vi "HEWH General Start End Draw.vi"(7 "Index Type":T1, 8 "error in (no error)":errorcluster, 10 "Draw Start":i32, 11 "UEF Calculated Values in":T2 {"Data Indexes"."15 sec after Draw Index" format="%#.2f"; "Data Indexes"."15 sec after Draw Timestamp" format="%#.2f"; "Data Indexes"."Test Start Timestamp" format="%.2f"; "Data Indexes"."Test End Timestamp" format="%.2f"; "Data Indexes"."T0 Timestamp" format="%.2f"; "Data Indexes"."Tsf Timestamp" format="%.2f"; "Data Indexes"."Tsu0 Timestamp" format="%.2f"; "Data Indexes"."Tmax1 Timestamp" format="%.2f"; "Data Indexes"."Draw Index Timestamp" format="%#.2f"; "Data Indexes"."Non-Draw Timestamp" format="%#.2f"; "Data Indexes"."Heating Timestamp" format="%#.2f"; "Data Indexes"."Start Energy (BTU-Gas)" format="%.6f"; "Data Indexes"."Start Watt Hours" format="%.6f"; "Static Data"."V - Volume of Wh (True)" format="%.5f"; "Static Data"."T-Ambinet Nominal (°F)" format="%.5f"; "Static Data"."T-Inlet Setpoint (°F)" format="%.5f"; "Static Data"."T-Wh Setpoint (°F)" format="%.5f"; "Sampled Data"."Qe (Wh)" format="%.5f"; "Sampled Data"."Tau stby2 (hr)" format="%.5f"; "Sampled Data"."Tastby2 (°F)" format="%.5f"; "Sampled Data"."Qf (BTU)" format="%.5f"; "Sampled Data"."Qe (BTU)" format="%.5f"; "Sampled Data"."Tmax1 (°F)" format="%.5f"; "Sampled Data"."T0 (°F)" format="%.5f"; "Sampled Data"."Qr (BTU)" format="%.5f"; "Sampled Data"."T 24(°F)" format="%.5f"; "Sampled Data"."T astby(°F)" format="%.5f"; "Sampled Data"."T tstby(°F)" format="%.5f"; "Sampled Data"."T su0(°F)" format="%.5f"; "Sampled Data"."T suf(°F)" format="%.5f"; "Sampled Data"."Tau stby_1 (hr)" format="%.5f"; "Sampled Data"."Qsuf (BTU)" format="%.5f"; "Sampled Data"."Qsu0 (BTU)" format="%.5f"; "Calculated Values"."Draw Bonus Volume (gal)" format="%.6f"; "Calculated Values"."Adjustment Factor" format="%.6f"; "Calculated Values"."T*avg_del(n-1)" format="%.6f"; "Calculated Values"."T*min(n-1)" format="%.6f"; "Calculated Values"."T*avg_del(n)" format="%.6f"; "Calculated Values"."Vn" format="%.6f"; "Calculated Values"."Qdm (BTU)" format="%.6f"; "Calculated Values"."QHWD (BTU)" format="%.6f"; "Calculated Values"."QHW (BTU)" format="%.6f"; "Calculated Values"."UEF" format="%.6f"; "Calculated Values"."QHW67 (BTU)" format="%.6f"; "Calculated Values"."Qda (BTU)" format="%.6f"; "Calculated Values"."Qd (BTU)" format="%.6f"; "Calculated Values"."Q (BTU)" format="%.6f"; "Calculated Values"."UA (BTU/(hr*F))" format="%.6f"; "Calculated Values"."Qhr (BTU/hr)" format="%.6f"; "Calculated Values"."Qstby (BTU)" format="%.6f"; "Calculated Values"."nu_r" format="%.6f"; "Calculated Values"."CpUEF (BTU/(lb*F))" format="%.6f"; "Calculated Values"."rho_nu (lb/gal)" format="%.6f"; "Calculated Values"."V1- Vol (Gal)" format="%.6f"; "Calculated Values"."M cluster mass removed (lb)" format="%.6f"; "Calculated Values"."Cp theoretical (BTU/(lbm °F))" format="%.6f"; "Calculated Values"."Tin1 - Mean Inlet 1st Cluster (°F)" format="%.6f"; "Calculated Values"."Tdel1-Mean Outlet 1st Cluster(°F)" format="%.6f"; "Calculated Values"."Cp 24 (BTU/(lb*F))" format="%.6f"; "Calculated Values"."Cp standby (BTU/(lb*F))" format="%.6f"; "Calculated Values"."Cp2 (BTU/(lb*F))" format="%.6f"; "Calculated Values"."Cp1 (BTU/(lb*F))" format="%.6f"; "Calculated Values"."rho 24 (lb/gal)" format="%.6f"; "Calculated Values"."rho standby (lb/gal)" format="%.6f"; "Calculated Values"."rho 2 (lb/gal)" format="%.6f"; "Calculated Values"."Density of cold water All (lbm/gal)" format="%#.3g"; "Calculated Values"."CpHW (BTU/(lbm °F))" format="%#.3g"; "Calculated Values"."Density of hot water All (lbm/gal)" format="%#.3g"; "Calculated Values"."Mass of water All (lbm)" format="%#.3f"}) -> (0 "error out":errorcluster, 2 "End Index":i32, 3 "UEF Calculated Values Output":T2 {"Data Indexes"."15 sec after Draw Index" format="%#.2f"; "Data Indexes"."15 sec after Draw Timestamp" format="%#.2f"; "Data Indexes"."Test Start Timestamp" format="%.2f"; "Data Indexes"."Test End Timestamp" format="%.2f"; "Data Indexes"."T0 Timestamp" format="%.2f"; "Data Indexes"."Tsf Timestamp" format="%.2f"; "Data Indexes"."Tsu0 Timestamp" format="%.2f"; "Data Indexes"."Tmax1 Timestamp" format="%.2f"; "Data Indexes"."Draw Index Timestamp" format="%#.2f"; "Data Indexes"."Non-Draw Timestamp" format="%#.2f"; "Data Indexes"."Heating Timestamp" format="%#.2f"; "Data Indexes"."Start Energy (BTU-Gas)" format="%.6f"; "Data Indexes"."Start Watt Hours" format="%.6f"; "Static Data"."V - Volume of Wh (True)" format="%.5f"; "Static Data"."T-Ambinet Nominal (°F)" format="%.5f"; "Static Data"."T-Inlet Setpoint (°F)" format="%.5f"; "Static Data"."T-Wh Setpoint (°F)" format="%.5f"; "Sampled Data"."Qe (Wh)" format="%.5f"; "Sampled Data"."Tau stby2 (hr)" format="%.5f"; "Sampled Data"."Tastby2 (°F)" format="%.5f"; "Sampled Data"."Qf (BTU)" format="%.5f"; "Sampled Data"."Qe (BTU)" format="%.5f"; "Sampled Data"."Tmax1 (°F)" format="%.5f"; "Sampled Data"."T0 (°F)" format="%.5f"; "Sampled Data"."Qr (BTU)" format="%.5f"; "Sampled Data"."T 24(°F)" format="%.5f"; "Sampled Data"."T astby(°F)" format="%.5f"; "Sampled Data"."T tstby(°F)" format="%.5f"; "Sampled Data"."T su0(°F)" format="%.5f"; "Sampled Data"."T suf(°F)" format="%.5f"; "Sampled Data"."Tau stby_1 (hr)" format="%.5f"; "Sampled Data"."Qsuf (BTU)" format="%.5f"; "Sampled Data"."Qsu0 (BTU)" format="%.5f"; "Calculated Values"."Draw Bonus Volume (gal)" format="%.6f"; "Calculated Values"."Adjustment Factor" format="%.6f"; "Calculated Values"."T*avg_del(n-1)" format="%.6f"; "Calculated Values"."T*min(n-1)" format="%.6f"; "Calculated Values"."T*avg_del(n)" format="%.6f"; "Calculated Values"."Vn" format="%.6f"; "Calculated Values"."Qdm (BTU)" format="%.6f"; "Calculated Values"."QHWD (BTU)" format="%.6f"; "Calculated Values"."QHW (BTU)" format="%.6f"; "Calculated Values"."UEF" format="%.6f"; "Calculated Values"."QHW67 (BTU)" format="%.6f"; "Calculated Values"."Qda (BTU)" format="%.6f"; "Calculated Values"."Qd (BTU)" format="%.6f"; "Calculated Values"."Q (BTU)" format="%.6f"; "Calculated Values"."UA (BTU/(hr*F))" format="%.6f"; "Calculated Values"."Qhr (BTU/hr)" format="%.6f"; "Calculated Values"."Qstby (BTU)" format="%.6f"; "Calculated Values"."nu_r" format="%.6f"; "Calculated Values"."CpUEF (BTU/(lb*F))" format="%.6f"; "Calculated Values"."rho_nu (lb/gal)" format="%.6f"; "Calculated Values"."V1- Vol (Gal)" format="%.6f"; "Calculated Values"."M cluster mass removed (lb)" format="%.6f"; "Calculated Values"."Cp theoretical (BTU/(lbm °F))" format="%.6f"; "Calculated Values"."Tin1 - Mean Inlet 1st Cluster (°F)" format="%.6f"; "Calculated Values"."Tdel1-Mean Outlet 1st Cluster(°F)" format="%.6f"; "Calculated Values"."Cp 24 (BTU/(lb*F))" format="%.6f"; "Calculated Values"."Cp standby (BTU/(lb*F))" format="%.6f"; "Calculated Values"."Cp2 (BTU/(lb*F))" format="%.6f"; "Calculated Values"."Cp1 (BTU/(lb*F))" format="%.6f"; "Calculated Values"."rho 24 (lb/gal)" format="%.6f"; "Calculated Values"."rho standby (lb/gal)" format="%.6f"; "Calculated Values"."rho 2 (lb/gal)" format="%.6f"; "Calculated Values"."Density of cold water All (lbm/gal)" format="%#.3g"; "Calculated Values"."CpHW (BTU/(lbm °F))" format="%#.3g"; "Calculated Values"."Density of hot water All (lbm/gal)" format="%#.3g"; "Calculated Values"."Mass of water All (lbm)" format="%#.3f"})   [LabVIEW 2023]
uses:
  Type Definitions/UEF Constants.ctl
  Type Definitions/HEWH Draw Stats.ctl
  Type Definitions/HEWH FHR Draw Type.ctl
  Type Definitions/FHR Bins.ctl
  Type Definitions/HEWH Meter Type.ctl
  Type Definitions/HEWH Index Type.ctl
panel:
  out "subarray":dbl[](array[numeric])
  # "FHR"
  # "FHR"
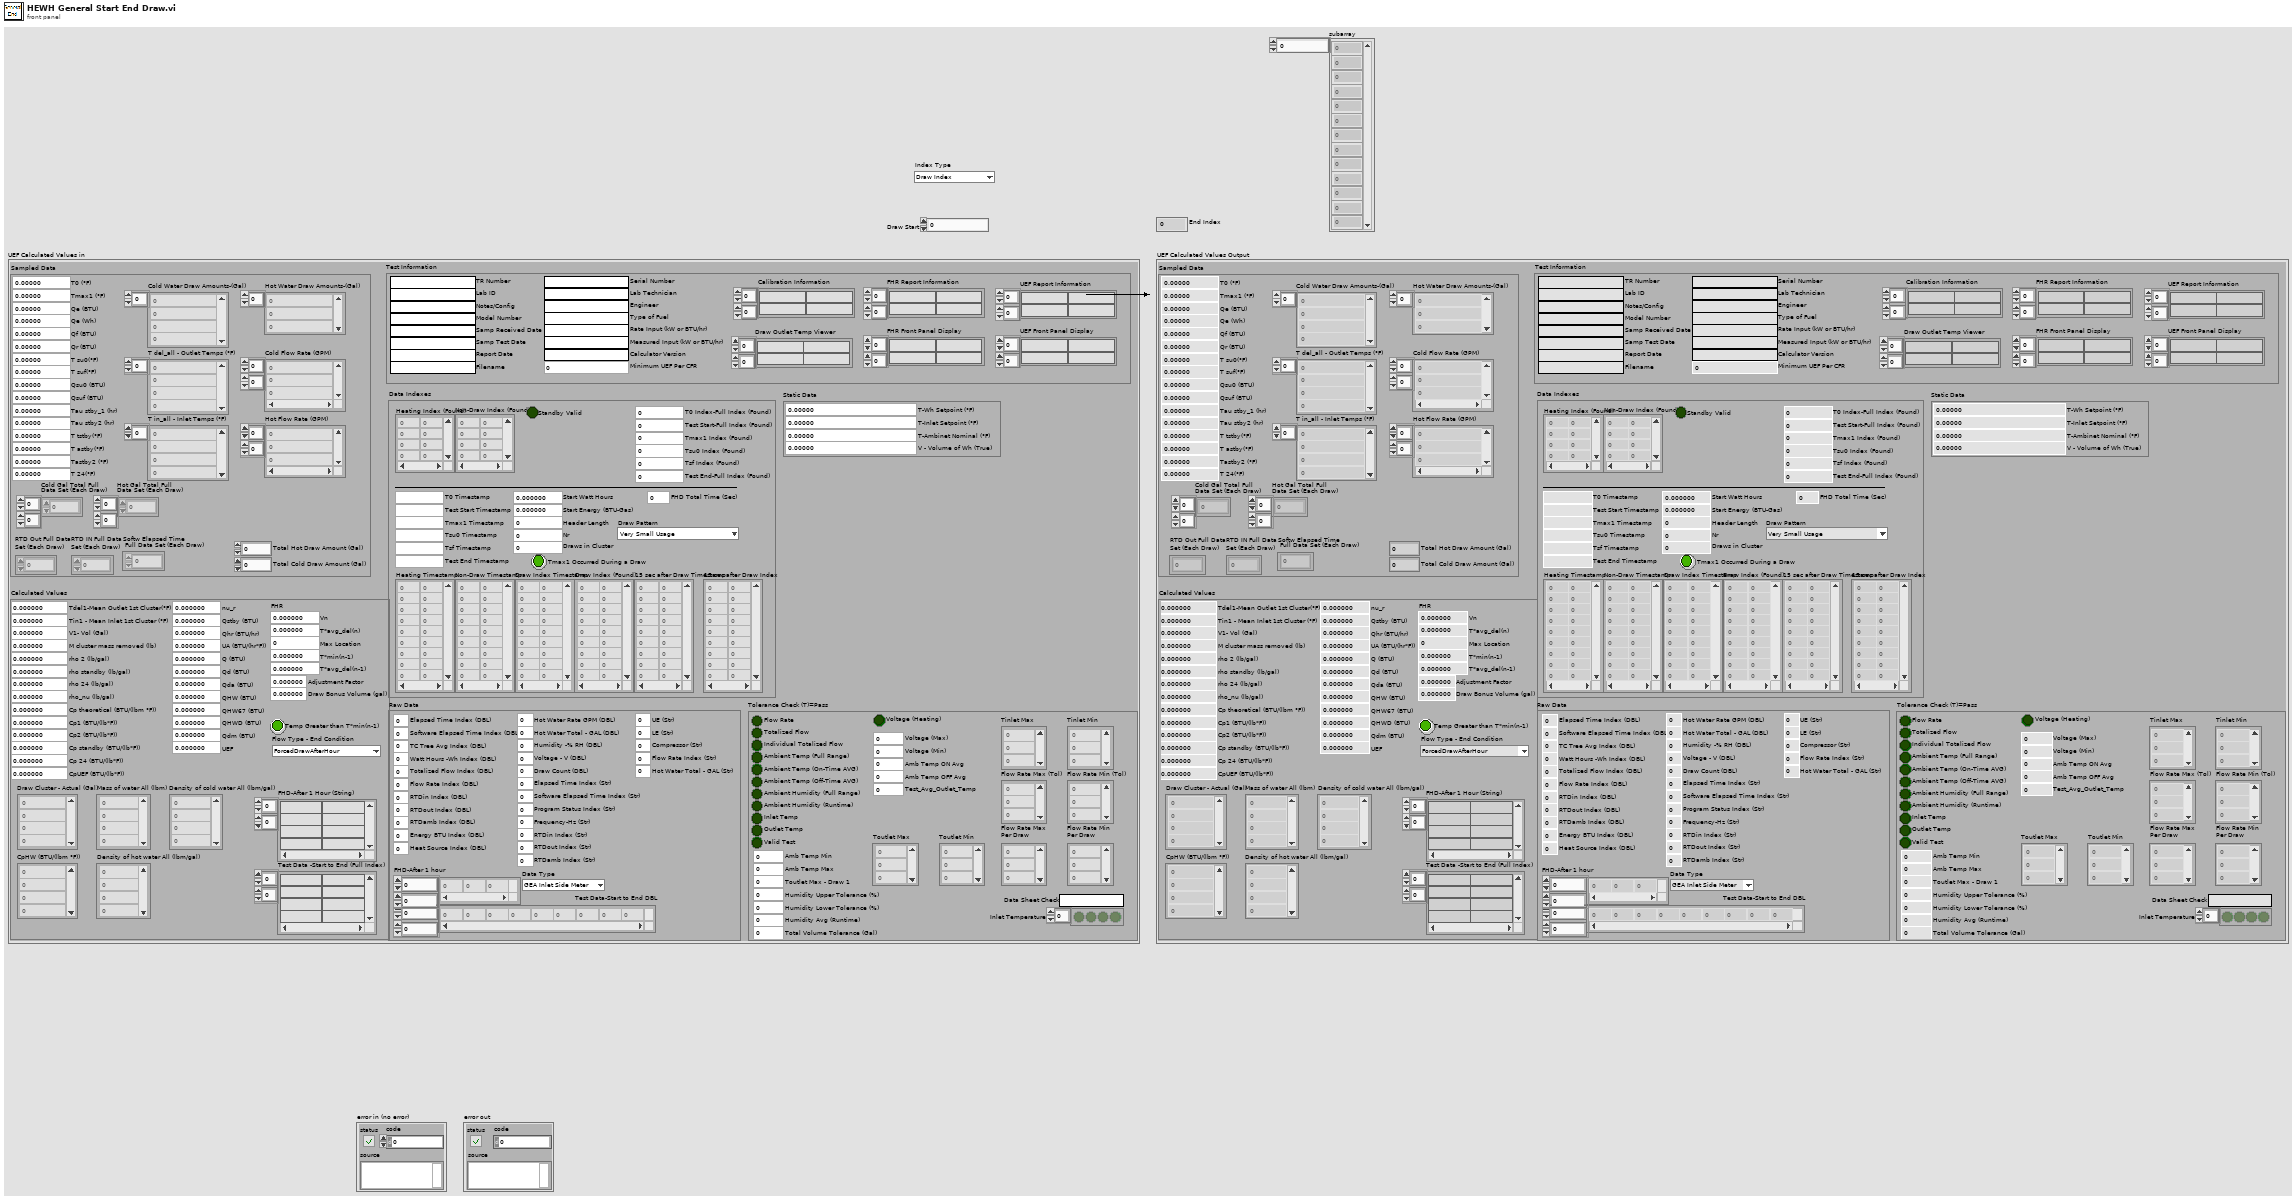
[diagram p1: front panel]
types:
  T1 = typedef "HEWH Index Type.ctl" = enum16{"Draw Index", "Heating Index", "Temp Based (FHD)"}
  T2 = typedef "UEF Constants.ctl" = cluster{"Calculated Values":T3, "Sampled Data":cluster{"Cold Water Draw Amounts-(Gal)":dbl[], "T del_all - Outlet Temps (°F)":dbl[], "T in_all - Inlet Temps (°F)":dbl[], "Qsu0 (BTU)":dbl, "Qsuf (BTU)":dbl, "Tau stby_1 (hr)":dbl, "T suf(°F)":dbl, "T su0(°F)":dbl, "T tstby(°F)":dbl, "T astby(°F)":dbl, "T 24(°F)":dbl, "Qr (BTU)":dbl, "T0 (°F)":dbl, "Tmax1 (°F)":dbl, "Qe (BTU)":dbl, "Qf (BTU)":dbl, "Tastby2 (°F)":dbl, "RTD Out Full Data\nSet (Each Draw)":dbl[][], "RTD IN Full Data\nSet (Each Draw)":dbl[][], "Tau stby2 (hr)":dbl, "Hot Water Draw Amounts-(Gal)":dbl[], "Cold Flow Rate (GPM)":dbl[][], "Hot Flow Rate (GPM)":dbl[][], "Softw Elapsed Time\n Full Data Set (Each Draw)":dbl[][], "Cold Gal Total Full\nData Set (Each Draw)":dbl[][], "Total Hot Draw Amount (Gal) ":dbl, "Total Cold Draw Amount (Gal)":dbl, "Qe (Wh)":dbl, "Hot Gal Total Full\nData Set (Each Draw)":dbl[][]}, "Static Data":cluster{"T-Wh Setpoint (°F)":dbl, "T-Inlet Setpoint (°F)":dbl, "T-Ambinet Nominal (°F)":dbl, "V - Volume of Wh (True)":dbl}, "Data Indexes":cluster{"Test Start-Full Index (Found)":i32, "Header Length":i32, "Draw Index (Found)":i32[][], "Nr":i32, "Start Watt Hours":dbl, "Tsu0 Index (Found)":i32, "Tsf Index (Found)":i32, "Start Energy (BTU-Gas)":dbl, "Draws in Cluster":i32, "T0 Index-Full Index (Found)":i32, "Non-Draw Index (Found)":i32[][], "Tmax1 Index (Found)":i32, "Test End-Full Index (Found)":i32, "Heating Index (Found)":i32[][], "Heating Timestamp":dbl[][], "Non-Draw Timestamp":dbl[][], "Draw Index Timestamp":dbl[][], "Tmax1 Timestamp":dbl, "Tsu0 Timestamp":dbl, "Tsf Timestamp":dbl, "T0 Timestamp":dbl, "Test End Timestamp":dbl, "Test Start Timestamp":dbl, "15 sec after Draw Timestamp":dbl[][], "15 sec after Draw Index":dbl[][], "Tmax1 Occurred During a Draw":bool, "FHD Total Time (Sec)":dbl, "Draw Pattern":T5, "Standby Valid":bool}, "Raw Data":cluster{"Elapsed Time Index (DBL)":i32, "Software Elapsed Time Index (DBL)":i32, "TC Tree Avg Index (DBL)":i32, "Watt Hours -Wh Index (DBL)":i32, "Energy BTU Index (DBL)":i32, "Totalized Flow Index (DBL)":i32, "Flow Rate Index (DBL)":i32, "Program Status Index (Str)":i32, "RTDin Index (DBL)":i32, "RTDout Index (DBL)":i32, "RTDamb Index (DBL)":i32, "Test Data-Start to End DBL":dbl[][], "Data Type":T6, "Heat Source Index (DBL)":i32, "Hot Water Rate GPM (DBL)":i32, "Hot Water Total - GAL (DBL)":i32, "FHD-After 1 hour":dbl[][], "Humidity -% RH (DBL)":i32, "Voltage - V (DBL)":i32, "Draw Count (DBL)":i32, "Elapsed Time Index (Str)":i32, "Software Elapsed Time Index (Str)":i32, "Frequency-Hz (Str)":i32, "RTDin Index (Str)":i32, "RTDout Index (Str)":i32, "RTDamb Index (Str)":i32, "UE (Str)":i32, "LE (Str)":i32, "Compressor (Str)":i32, "Flow Rate Index (Str)":i32, "Hot Water Total - GAL (Str)":i32}, "Tolerance Check (T)=Pass":cluster{"Flow Rate":bool, "Totalized Flow":bool, "Ambient Temp (Full Range)":bool, "Ambient Humidity (Full Range)":bool, "Inlet Temp":bool, "Outlet Temp":bool, "Valid Test":bool, "Individual Totalized Flow":bool, "Data Sheet Check":string, "Inlet Temperature":bool[], "Tinlet Max":dbl[], "Tinlet Min":dbl[], "Flow Rate Max (Tol)":dbl[], "Flow Rate Min (Tol)":dbl[], "Amb Temp Max":dbl, "Amb Temp Min":dbl, "Toutlet Max - Draw 1":dbl, "Humidity Upper Tolerance (%)":dbl, "Total Volume Tolerance (Gal)":dbl, "Humidity Lower Tolerance (%)":dbl, "Flow Rate Max\nPer Draw":dbl[], "Flow Rate Min\nPer Draw":dbl[], "Ambient Humidity (Runtime)":bool, "Humidity Avg (Runtime)":dbl, "Ambient Temp (On-Time AVG)":bool, "Ambient Temp (Off-Time AVG)":bool, "Amb Temp OFF Avg":dbl, "Amb Temp ON Avg":dbl, "Voltage (Heating)":bool, "Voltage (Min)":dbl, "Voltage (Max)":dbl, "Toutlet Max":dbl[], "Toutlet Min":dbl[], "Test_Avg_Outlet_Temp":dbl}, "Test Information":cluster{"TR Number":string, "Lab ID":string, "Notes/Config":string, "Model Number":string, "Serial Number":string, "Lab Technician":string, "Engineer":string, "Type of Fuel":string, "Samp Received Date":string, "Samp Test Date":string, "Report Date":string, "Rate Input (kW or BTU/hr)":string, "Measured Input (kW or BTU/hr)":string, "Filename":string, "Calibration Information":string[][], "Calculator Version":string, "Minimum UEF Per CFR":dbl, "UEF Report Information":string[][], "FHR Report Information":string[][], "FHR Front Panel Display":string[][], "UEF Front Panel Display":string[][], "Draw Outlet Temp Viewer":string[][]}}
  T3 = typedef "HEWH Draw Stats.ctl" = cluster{"Draw Cluster - Actual (Gal)":dbl[], "Mass of water All (lbm)":dbl[], "Density of hot water All (lbm/gal)":dbl[], "CpHW (BTU/(lbm °F))":dbl[], "rho 2 (lb/gal)":dbl, "rho standby (lb/gal)":dbl, "rho 24 (lb/gal)":dbl, "Cp1 (BTU/(lb*F))":dbl, "Cp2 (BTU/(lb*F))":dbl, "Cp standby (BTU/(lb*F))":dbl, "Cp 24 (BTU/(lb*F))":dbl, "nu_r":dbl, "Qstby (BTU)":dbl, "Qhr (BTU/hr)":dbl, "UA (BTU/(hr*F))":dbl, "Q (BTU)":dbl, "Qd (BTU)":dbl, "Qda (BTU)":dbl, "QHW67 (BTU)":dbl, "UEF":dbl, "Tdel1-Mean Outlet 1st Cluster(°F)":dbl, "Tin1 - Mean Inlet 1st Cluster (°F)":dbl, "Cp theoretical (BTU/(lbm °F))":dbl, "M cluster mass removed (lb)":dbl, "V1- Vol (Gal)":dbl, "Test Data -Start to End (Full Index)":string[][], "rho_nu (lb/gal)":dbl, "Density of cold water All (lbm/gal)":dbl[], "CpUEF (BTU/(lb*F))":dbl, "QHW (BTU)":dbl, "QHWD (BTU)":dbl, "Qdm (BTU)":dbl, "FHD-After 1 Hour (String)":string[][], "Vn":dbl, "T*avg_del(n)":dbl, "Max Location":i32, "T*min(n-1)":dbl, "T*avg_del(n-1)":dbl, "Temp Greater than T*min(n-1)":bool, "Adjustment Factor":dbl, "Draw Bonus Volume (gal)":dbl, "Flow Type - End Condition":T4}
  T4 = typedef "HEWH FHR Draw Type.ctl" = enum16{"ForcedDrawAfterHour", "HeatingCutoffBeforeHour"}
  T5 = typedef "FHR Bins.ctl" = enum16{"Very Small Usage", "Low Usage", "Medium Usage", "High Usage", "Undefined"}
  T6 = typedef "HEWH Meter Type.ctl" = enum16{"GEA Inlet Side Meter", "GEA Outlet Side Meter", "CSA Inlet Side Meter"}
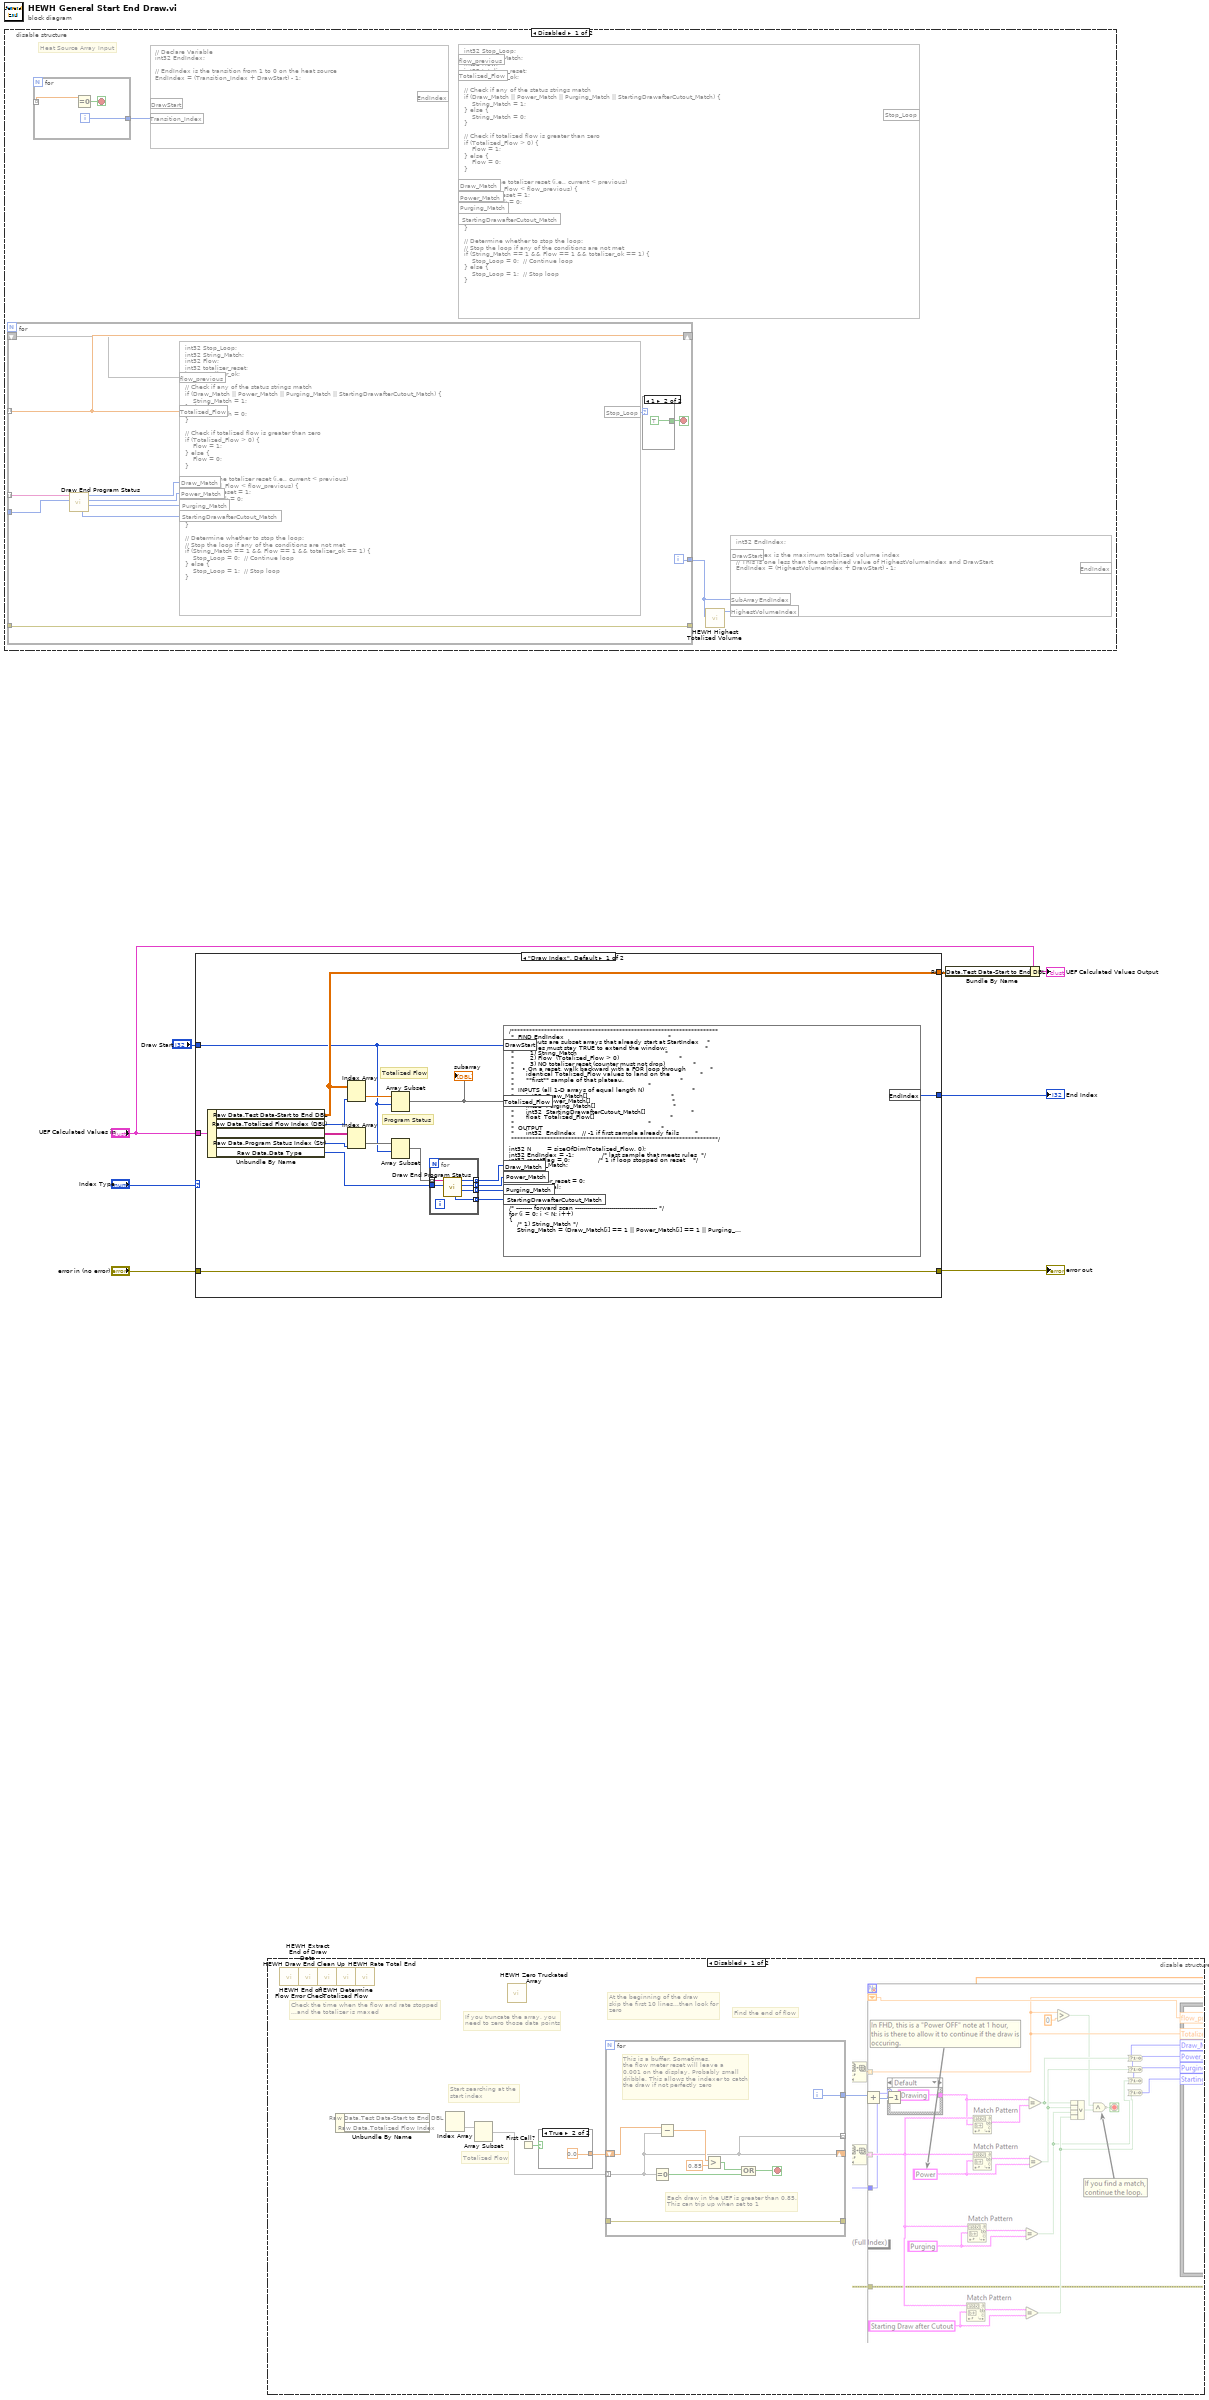
[diagram p0: block diagram]
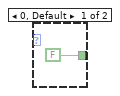
[diagram p2: hidden frame]
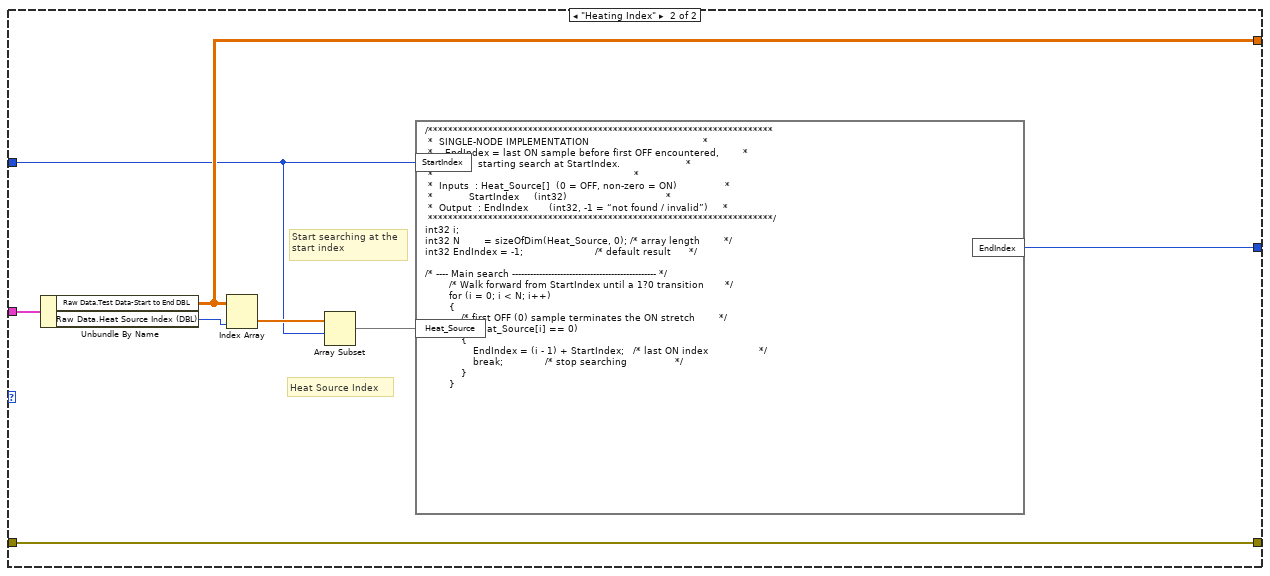
[diagram p6: hidden frame]
diagram:
  n1 = disable-structure shown="Disabled" {
    frame Disabled {
      # "Heat Source Array Input"
      n2 = for {
        tunnel: [w23] -> w9
        tunnel: _ -> [w20] mode=indexing
        tunnel: _ -> [w22]
        tunnel: [w22] -> _
        tunnel: _ -> [w21]
        tunnel: _ -> [w13] mode=indexing
        shift-right: [w13] -> _
        shift-left: _ -> [w12]
        i -> [w23]
        stop <- w14 stop-if-true
        n3 = call "Draw End Program Status.vi"("Data Type"=w21, "Program Status String"=w20) -> ("Purging_Match"=w18:i16, "Power_Match"=w16:i16, "Draw_Match"=w19:i16, "StartingDrawafterCutout_Match"=w17:i16)  [unwired: 6 in]
        n4 = formula code="int32 Stop_Loop;\nint32 String_Match;\nint32 Flow;\nint32 totalizer_reset;\nint32 totalizer_ok;\n\n// Check if any of the status strings match\nif (Draw_Match || Power_Match || Purging_Match || StartingDrawafterCutout_Match) {\n    String_Match = 1;\n} else {\n    String_Match = 0;\n}\n\n// Check if totalized flow is greater than zero\nif (Totalized_Flow > 0) {\n    Flow = 1;\n} else {\n    Flow = 0;\n}\n\n// Check if the totalizer reset (i.e., current < previous)\nif (Totalized_Flow < flow_previous) {\n    totalizer_reset = 1;\n    totalizer_ok = 0;\n} else {\n    totalizer_reset = 0;\n    totalizer_ok = 1;\n}\n\n// Determine whether to stop the loop:\n// Stop the loop if any of the conditions are not met\nif (String_Match == 1 && Flow == 1 && totalizer_ok == 1) {\n    Stop_Loop = 0;  // Continue loop\n} else {\n    Stop_Loop = 1;  // Stop loop\n}"("Draw_Match"=w19, "Power_Match"=w16, "Purging_Match"=w18, "StartingDrawafterCutout_Match"=w17, "Totalized_Flow"=w13, "flow_previous"=w12) -> ("Stop_Loop"=w15:i32)
        n5 = case shown="1" w15 {
          tunnel: [FALSE TRUE] -> w14
          frame 0, Default {
          }
          frame 1 {
          }
        }
      }
      n6 = for {
        tunnel: _ -> [w28] mode=indexing
        tunnel: [w26] -> w11
        i -> [w26]
        stop <- w27 stop-if-true
        n7 = Equal To 0?(x=w28) -> (x = 0?=w27:bool)
      }
      n8 = formula code="// Declare Variable\nint32 EndIndex;\n\n// EndIndex is the transition from 1 to 0 on the heat source\nEndIndex = (Transition_Index + DrawStart) - 1;"("Transition_Index"=w11) -> ()  [unwired: 1 in, 1 out]
      n9 = formula code="int32 Stop_Loop;\nint32 String_Match;\nint32 Flow;\nint32 totalizer_reset;\nint32 totalizer_ok;\n\n// Check if any of the status strings match\nif (Draw_Match || Power_Match || Purging_Match || StartingDrawafterCutout_Match) {\n    String_Match = 1;\n} else {\n    String_Match = 0;\n}\n\n// Check if totalized flow is greater than zero\nif (Totalized_Flow > 0) {\n    Flow = 1;\n} else {\n    Flow = 0;\n}\n\n// Check if the totalizer reset (i.e., current < previous)\nif (Totalized_Flow < flow_previous) {\n    totalizer_reset = 1;\n    totalizer_ok = 0;\n} else {\n    totalizer_reset = 0;\n    totalizer_ok = 1;\n}\n\n// Determine whether to stop the loop:\n// Stop the loop if any of the conditions are not met\nif (String_Match == 1 && Flow == 1 && totalizer_ok == 1) {\n    Stop_Loop = 0;  // Continue loop\n} else {\n    Stop_Loop = 1;  // Stop loop\n}"() -> ()  [unwired: 6 in, 1 out]
      n10 = call "HEWH Highest Totalized Volume.vi"("Sub Array End Index in"=w9) -> ("Highest Volume Index"=w10:i32)  [unwired: 9 in, 1 out]
      n11 = formula code="int32 EndIndex;\n\n// EndIndex is the maximum totalized volume index\n// This is one less than the combined value of HighestVolumeIndex and DrawStart\nEndIndex = (HighestVolumeIndex + DrawStart) - 1;"("HighestVolumeIndex"=w10, "SubArrayEndIndex"=w9) -> ()  [unwired: 1 in, 1 out]
    }
    frame Enabled {
    }
  }
  n12 = case shown="\"Draw Index\", Default" "Index Type" {
    tunnel: "UEF Calculated Values in" -> [w45 w59]
    tunnel: [w39 w57] -> w2
    tunnel: "Draw Start" -> [w31 w54]
    tunnel: "error in (no error)" -> [w29 w56]
    tunnel: [w29 w56] -> w1
    tunnel: [w30 w52] -> w3
    frame "Draw Index", Default {
      # "Program Status"
      # "Totalized Flow"
      n13 = Unbundle By Name(w45) -> ("Raw Data.Test Data-Start to End DBL"=w39:dbl[][], "Raw Data.Totalized Flow Index (DBL)"=w40:i32, "Calculated Values.Test Data -Start to End (Full Index)"=w42:string[][], "Raw Data.Program Status Index (Str)"=w41:i32, "Raw Data.Data Type"=w37:T6)
      n14 = Index Array(array=w39, index (col)=w40) -> (element=w44:dbl[])  [unwired: 1 in]
      n15 = Index Array(array=w42, index (col)=w41) -> (element=w43:string[])  [unwired: 1 in]
      n16 = Array Subset(array=w44, index=w31) -> (w36:dbl[])  [unwired: 1 in]
      "subarray" <- w36
      n17 = Array Subset(array=w43, index=w31) -> (w38:string[])  [unwired: 1 in]
      n18 = for {
        tunnel: w38 -> [w51] mode=indexing
        tunnel: w37 -> [w50]
        tunnel: [w49] -> w35 mode=indexing
        tunnel: [w48] -> w34 mode=indexing
        tunnel: [w47] -> w33 mode=indexing
        tunnel: [w46] -> w32 mode=indexing
        n19 = call "Draw End Program Status.vi"("Data Type"=w50, "Program Status String"=w51) -> ("Purging_Match"=w47:i16, "Power_Match"=w48:i16, "Draw_Match"=w49:i16, "StartingDrawafterCutout_Match"=w46:i16)  [unwired: 6 in]
      }
      n20 = formula code="/*********************************************************************\n *  FIND EndIndex                                                    *\n *    • Inputs are subset arrays that already start at StartIndex    *\n *    • Rules must stay TRUE to extend the window:                   *\n *        1) String_Match                                            *\n *        2) Flow  (Totalized_Flow > 0)                              *\n *        3) NO totalizer reset (counter must not drop)              *\n *    • On a reset, walk backward with a FOR loop through            *\n *      identical Totalized_Flow values to land on the               *\n *      **first** sample of that plateau.                            *\n *                                                                   *\n *  INPUTS (all 1-D arrays of equal length N)                        *\n *      int32  Draw_Match[]                                          *\n *      int32  Power_Match[]                                         *\n *      int32  Purging_Match[]                                       *\n *      int32  StartingDrawafterCutout_Match[]                       *\n *      float  Totalized_Flow[]                                      *\n *                                                                   *\n *  OUTPUT                                                           *\n *      int32  EndIndex   // -1 if first sample already fails        *\n *********************************************************************/\n\nint32 N        = sizeOfDim(Totalized_Flow, 0);\nint32 EndIndex = -1;              /* last sample that meets rules  */\nint32 resetFlag = 0;              /* 1 if loop stopped on reset    */\nint32 String_Match;\nint32 i, j;\nint32 Flow;\nint32 totalizer_reset = 0;\nfloat plateauVal;\nfloat Absolute;\nint32 earliestIdx;\n\n/* -------- forward scan ----------------------------------------- */\nfor (i = 0; i < N; i++)\n{\n    /* 1) String_Match */\n    String_Match = (Draw_Match[i] == 1 || Power_Match[i] == 1 || Purging_Match[i] == 1 || StartingDrawafterCutout_Match[i] == 1) ? 1 : 0;\n\n    /* 2) Flow present */\n    Flow = (Totalized_Flow[i] > 0.0) ? 1 : 0;\n    Absolute = Totalized_Flow[i];\n\n    if (i > 0)\n    {\n        /* 3a) Counter dropped */\n        if (Totalized_Flow[i] < Totalized_Flow[i - 1])\n         {   \n            totalizer_reset = 1;\n         }\n        /* 3b) Draw to Purge hand-off: prev {1,0}  to  curr {0,1}      */\n        else if (Draw_Match[i - 1]  == 1 && Purging_Match[i - 1] == 0 && Draw_Match[i] == 0 && Purging_Match[i] == 1)\n         { \n            totalizer_reset = 1;\n         }\n    }\n\n    /* ---- keep window open only if ALL rules true --------------- */\n    if (String_Match == 1 && Flow == 1 && totalizer_reset == 0)\n    {\n        EndIndex = i;            /* extend window */\n    }\n    else                         /* first failure */\n    {\n        if (totalizer_reset == 1)\n        {\n            EndIndex  = i - 1;   /* last good sample  */\n            resetFlag = 1;       /* remember cause    */\n        }\n        break;                   /* stop scanning     */\n    }\n}\n\n/* -------- backward FOR loop to earliest plateau sample ---------- */\nif (resetFlag == 1 && EndIndex >= 0)\n{\n    plateauVal = Totalized_Flow[EndIndex];\n    earliestIdx  = EndIndex;        /* start with last good */\n\n   /* Walk back while the value stays equal to plateauVal */\n    for (j = EndIndex - 1; j >= 0; j--)\n    {\n        if (Totalized_Flow[j] == plateauVal)\n        {\n            earliestIdx = j;              /* shift anchor back */\n        }\n        else\n        {\n            break;                        /* left the plateau  */\n        }\n    }\n\n    /* Convert subset index ? full-array index */\n    EndIndex = earliestIdx + DrawStart;\n}\nelse\n{\n    /* No reset or EndIndex < 0 ? just offset if valid           */\n    if (EndIndex >= 0)\n     {\n        EndIndex = EndIndex + DrawStart;\n     }\n}"("Draw_Match"=w35, "Power_Match"=w34, "Purging_Match"=w33, "StartingDrawafterCutout_Match"=w32, "Totalized_Flow"=w36, "DrawStart"=w31) -> ("EndIndex"=w30:i32)
    }
    frame "Heating Index" {
      # "Heat Source Index"
      # "Start searching at the \nstart index"
      n21 = Unbundle By Name(w59) -> ("Raw Data.Test Data-Start to End DBL"=w57:dbl[][], "Raw Data.Heat Source Index (DBL)"=w58:i32)
      n22 = Index Array(array=w57, index (col)=w58) -> (element=w55:dbl[])  [unwired: 1 in]
      n23 = Array Subset(array=w55, index=w54) -> (w53:dbl[])  [unwired: 1 in]
      n24 = formula code="/*********************************************************************\n *  SINGLE-NODE IMPLEMENTATION                                      *\n *    EndIndex = last ON sample before first OFF encountered,        *\n *               starting search at StartIndex.                      *\n *                                                                   *\n *  Inputs  : Heat_Source[]  (0 = OFF, non-zero = ON)                *\n *            StartIndex     (int32)                                 *\n *  Output  : EndIndex       (int32, -1 = “not found / invalid”)     *\n *********************************************************************/\nint32 i;\nint32 N        = sizeOfDim(Heat_Source, 0); /* array length        */\nint32 EndIndex = -1;                        /* default result      */\n\n/* ---- Main search ------------------------------------------------ */\n        /* Walk forward from StartIndex until a 1?0 transition       */\n        for (i = 0; i < N; i++)\n        {\n            /* first OFF (0) sample terminates the ON stretch        */\n            if (Heat_Source[i] == 0)\n            {\n                EndIndex = (i - 1) + StartIndex;   /* last ON index                 */\n                break;              /* stop searching                */\n            }\n        }"("Heat_Source"=w53, "StartIndex"=w54) -> ("EndIndex"=w52:i32)
    }
  }
  "End Index" <- w3
  "error out" <- w1
  n25 = disable-structure shown="Disabled" {
    frame Disabled {
      # "If you truncate the array, you\nneed to zero those data points"
      # "Totalized Flow"
      # "Start searching at the \nstart index"
      # "Find the end of flow"
      # "At the beginning of the draw\nskip the first 10 lines...then look for\nzero"
      # "Check the time when the flow and rate stopped\n...and the totalizer is maxed"
      n26 = call "HEWH End of Flow Error Check.vi"() -> ()  [unwired: 10 in, 2 out]
      n27 = call "HEWH Extract End of Draw Data.vi"() -> ()  [unwired: 8 in, 4 out]
      n28 = call "HEWH Draw End Clean Up.vi"() -> ()  [unwired: 13 in, 3 out]
      n29 = Unbundle By Name() -> ()  [unwired: 1 in, 2 out]
      n30 = call "HEWH Determine Totalized Flow.vi"() -> ()  [unwired: 12 in, 4 out]
      n31 = call "HEWH Rate Total End.vi"() -> ()  [unwired: 14 in, 2 out]
      n32 = Index Array() -> (element=w62)  [unwired: 3 in]
      n33 = Array Subset(array=w62) -> (w63:void[])  [unwired: 2 in]
      n34 = call "HEWH Zero Truckated Array.vi"() -> ()  [unwired: 10 in, 2 out]
      n35 = First Call?() -> (First Call?: T/F=w61:bool)
      n36 = case shown="True" w61 {
        tunnel: [_ 0.0] -> w60
        frame False {
        }
        frame True {
        }
      }
      n37 = for {
        tunnel: w63 -> [w71] mode=indexing
        tunnel: [w75] -> w65
        shift-right: [w71] -> _
        shift-left: w60 -> [w74]
        tunnel: [w71] -> _ mode=indexing
        tunnel: _ -> [w70]
        tunnel: [w70] -> _
        i -> [w75]
        stop <- w67 stop-if-true
        # "This is a buffer. Sometimes,\nthe flow meter reset will leave a \n0.001 on the display. Probably small\ndribble. This allows the indexer to catch\nthe draw if not perfectly zero"
        # "Each draw in the UEF is greater than 0.85. \nThis can trip up when set to 1"
        n38 = Equal To 0?(x=w71) -> (x = 0?=w68:bool)
        n39 = Subtract(x=w74, y=w71) -> (x-y=w72:dbl)
        n40 = Greater?(x=w72, y=0.85) -> (0:w69:bool)
        n41 = Compound Arithmetic op=OR(w69, w68) -> (w67:bool)
      }
      n42 = Add(x=w65) -> (x+y=w64:i32)  [unwired: 1 in]
      n43 = Decrement(x=w64) -> ()  [unwired: 1 out]
    }
    frame Enabled {
    }
  }
  n44 = Bundle By Name(cluster="UEF Calculated Values in", "Raw Data.Test Data-Start to End DBL"=w2) -> (→"UEF Calculated Values Output":T2)
